vi "Create_folder_if_doesnt_exist.vi"(8 "error in (no error)":errorcluster, 11 "Folder name in":path) -> (0 "error out":errorcluster, 3 "Folder out":path)   [LabVIEW 2012]
panel:
  out "file or folder exists?":bool
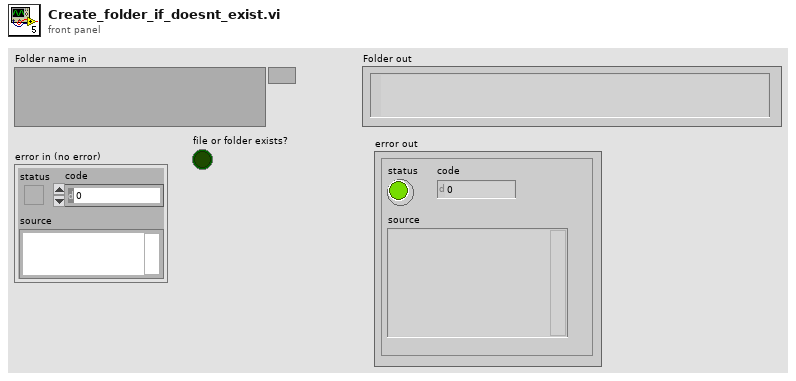
[diagram p1: front panel]
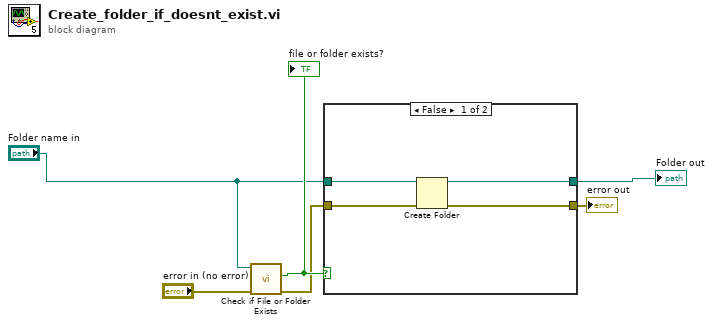
[diagram p0: block diagram]
diagram:
  n1 = call <vilib>:"Check if File or Folder Exists.vi"("error in (no error)"="error in (no error)", "path"="Folder name in") -> ("error out"=w3:errorcluster, "file or folder exists?"=w6:bool)  [unwired: 7 in, 1 out]
  "file or folder exists?" <- w6
  n2 = case shown="False" w6 {
    tunnel: "Folder name in" -> [w10 w12]
    tunnel: [w9 w12] -> w4
    tunnel: w3 -> [w8 w11]
    tunnel: [w7 w11] -> w2
    frame False {
      n3 = Create Folder(path (use dialog)=w10, error in=w8) -> (created path=w9:path, error out=w7:errorcluster)  [unwired: 1 in, 1 out]
    }
    frame True {
    }
  }
  "Folder out" <- w4
  "error out" <- w2
